vi "离线起止通道.vi"(8 "错误输入":errorcluster caption="输出簇", 11 "文件句柄":i32) -> (0 "错误输出":errorcluster, 1 "终止通道":i32, 2 "起始通道":i32, 3 "文件句柄出":i32, 5 "通道数量":i32)   [LabVIEW 2011]
uses:
  dll/em9636.dll
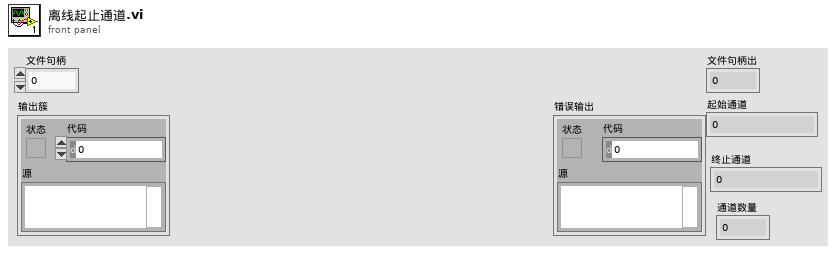
[diagram p1: front panel]
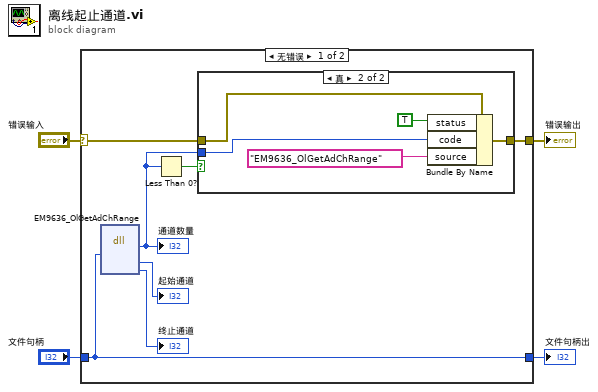
[diagram p0: block diagram]
diagram:
  n1 = case shown="无错误" "错误输入" {
    selector: "错误输入" -> [w7 w19]
    tunnel: [w9 w19] -> w3
    tunnel: "文件句柄" -> [w8 w18]
    tunnel: [w8 w18] -> w1
    frame No Error {
      n2 = dll-call lib="PTH1abs Eèµ éç LABVIEWæºVI(v2.0)EM9636BD)EM9636BDè°ç¨APIå½æ°æ¹æ³éè®¯ä¾ç¨EM9636labview8.5-1511048.5dll\nem9636.dll" fn="EM9636_OlGetAdChRange"("文件句柄"=w8) -> ("通道数量"=w10:i32, "起始通道"=→"起始通道":i32, "终止通道"=→"终止通道":i32)  [unwired: 6 in, 2 out]
      "通道数量" <- w10
      n3 = Less Than 0?(x=w10) -> (x < 0?=w11:bool)
      n4 = case shown="真" w11 {
        tunnel: [w12 w15] -> w9
        tunnel: w7 -> [w12 w17]
        tunnel: w10 -> [_ w14]
        frame False {
        }
        frame True {
          n5 = Bundle By Name(cluster=w17, "status"=TRUE, "code"=w14, "source"="EM9636_OlGetAdChRange") -> (w15:errorcluster)
        }
      }
    }
    frame Error {
    }
  }
  "文件句柄出" <- w1
  "错误输出" <- w3
